vi "PlotSimSharpness.vi"(1 "StepSize":dbl format="%#_13g", 2 "Focus Parameters":T1, 3 "Range Z":dbl format="%#_13g") -> (0 "Cluster":cluster{dbl[], dbl[]})   [LabVIEW 2014]
panel:
  # "LICENSED MATERIALS – PROPERTY OF IBM\nCopyright IBM Corp. 2016, 2016\nALL RIGHTS RESERVED"
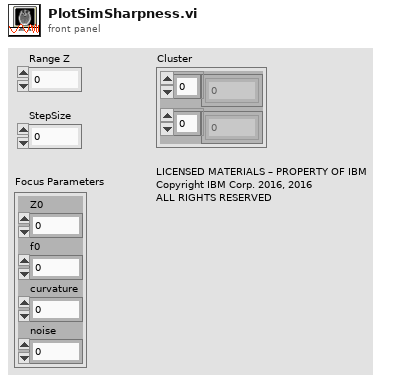
[diagram p1: front panel]
types:
  T1 = cluster{"Z0":dbl, "f0":dbl, "curvature":dbl, "noise":dbl}
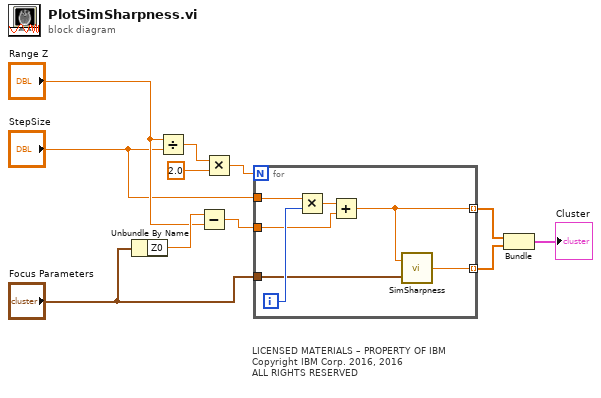
[diagram p0: block diagram]
diagram:
  # "LICENSED MATERIALS – PROPERTY OF IBM\nCopyright IBM Corp. 2016, 2016\nALL RIGHTS RESERVED"
  n1 = Unbundle By Name("Focus Parameters") -> ("Z0"=w11:dbl)
  n2 = Divide(x="Range Z", y="StepSize") -> (x/y=w1:dbl)
  n3 = Subtract(x=w11, y="Range Z") -> (x-y=w6:dbl)
  n4 = Multiply(x=w1, y=2.0) -> (x*y=w2:dbl)
  n5 = for {
    N: w2 -> [_]
    tunnel: "StepSize" -> [w18]
    tunnel: w6 -> [w15]
    tunnel: [w14] -> w7 mode=indexing
    tunnel: [w13] -> w8 mode=indexing
    tunnel: "Focus Parameters" -> [w12]
    i -> [w17]
    n6 = Multiply(x=w18, y=w17) -> (x*y=w16:dbl)
    n7 = Add(x=w16, y=w15) -> (x+y=w14:dbl)
    n8 = call "SimSharpness.vi"("Focus Parameters"=w12, "Z"=w14) -> ("Sharpness"=w13:dbl)
  }
  n9 = Bundle(w7, w8) -> (→"Cluster":cluster{dbl[], dbl[]})  [unwired: 1 in]
